vi "Configure Pattern Trigger Source.vi"(0 "VISA resource name":refnum<visa-resource-name>, 1 "Data Value (0)":i32, 5 "Trigger Source (20: None)":u16(ring)=20 items=["Channel 1", "Channel 2", "Channel 3", "Channel 4", "DIG 0", "DIG 1", "DIG 2", "DIG 3", "DIG 4", "DIG 5", "DIG 6", "DIG 7", "DIG 8", "DIG 9", "DIG 10", "DIG 11", "DIG 12", "DIG 13", "DIG 14", "DIG 15", "None"], 9 "Slope (0: Positive)":u16(ring) items=["Positive", "Negative"], 11 "error in (no error)":errorcluster, 12 "Data Mask (0)":i32) -> (4 "VISA resource name out":refnum<visa-resource-name>, 15 "error out":errorcluster)   [LabVIEW 2017, in "Agilent 6000 Series.lvlib"]
doc: "This VI configures the pattern trigger."
uses:
  <instrlib>/Agilent 6000 Series/Agilent 6000 Series.lvlib
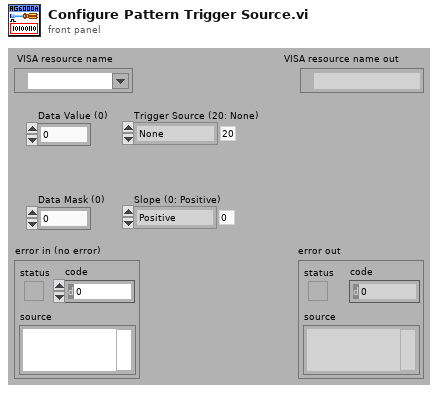
[diagram p1: front panel]
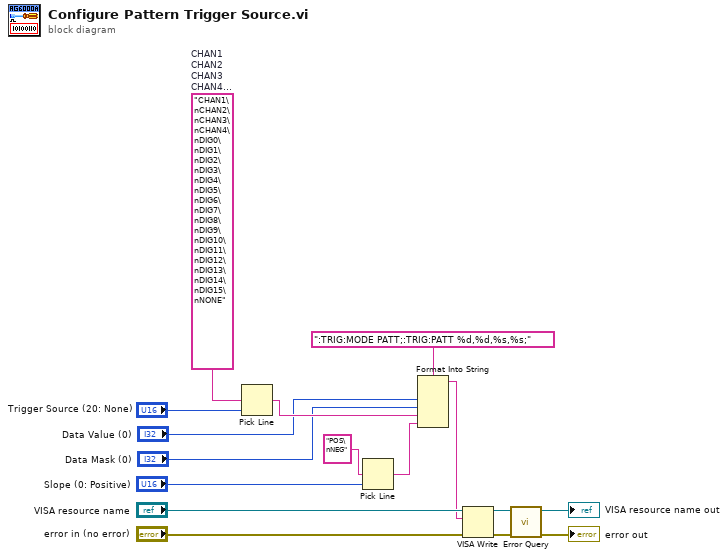
[diagram p0: block diagram]
diagram:
  w8 = "CHAN1\nCHAN2\nCHAN3\nCHAN4\nDIG0\nDIG1\nDIG2\nDIG3\nDIG4\nDIG5\nDIG6\nDIG7\nDIG8\nDIG9\nDIG10\nDIG11\nDIG12\nDIG13\nDIG14\nDIG15\nNONE"  # CHAN1 CHAN2 CHAN3 CHAN4 DIG0 DIG1 DIG2 DIG3 DIG4 DIG5 DIG6 DIG7 DIG8 DIG9 DIG10 DIG11 DIG12 DIG13 DIG14 DIG15 NONE
  n1 = Pick Line(multi-line string=w8, line index="Trigger Source (20: None)") -> (output string=w4:string)  [unwired: 1 in]
  n2 = Pick Line(multi-line string="POS\nNEG" ("Slope Command"), line index="Slope (0: Positive)") -> (output string=w5:string)  [unwired: 1 in]
  n3 = Format Into String(format string=":TRIG:MODE PATT;:TRIG:PATT %d,%d,%s,%s;" ("Source Command"), "Data Value (0)", "Data Mask (0)", w4, w5) -> (resulting string=w1:string)  [unwired: 2 in, 1 out]
  n4 = VISA Write(VISA resource name="VISA resource name", write buffer=w1, error in (no error)="error in (no error)") -> (VISA resource name out=w12:refnum<visa-resource-name>, error out=w11:errorcluster)  [unwired: 1 out]
  n5 = call <instrlib>:"Error Query.vi"("error in (no error)"=w11, "VISA resource name"=w12) -> ("error out"=→"error out":errorcluster, "VISA resource name out"=→"VISA resource name out":refnum<visa-resource-name>)  [unwired: 6 in, 2 out]
